vi "resolve VI reference.vi"(8 "error in":errorcluster, 10 "VI name":string, 11 "VI reference":refnum<vi>) -> (0 "error out":errorcluster, 3 "UI Ref":refnum<vi>)   [LabVIEW 2013, in "UI Reference runtime.lvclass"]
uses:
  UI Reference runtime.lvclass
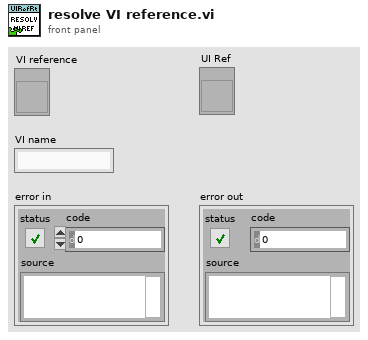
[diagram p1: front panel]
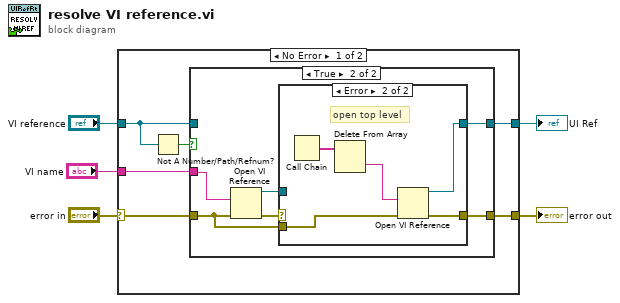
[diagram p0: block diagram]
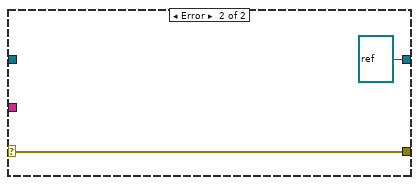
[diagram p4: hidden frame]
diagram:
  n1 = case shown="No Error" "error in" {
    selector: "error in" -> [w6 w28]
    tunnel: "VI reference" -> [w10 _]
    tunnel: [w9 refnum<vi> refnum ("VI reference")] -> w4
    tunnel: "VI name" -> [w8 _]
    tunnel: [w7 w28] -> w2
    frame No Error {
      n2 = Not A Number/Path/Refnum?(number/path/refnum=w10) -> (NaN/Path/Refnum?=w11:bool)
      n3 = case shown="True" w11 {
        tunnel: w10 -> [w13 _]
        tunnel: [w13 w17] -> w9
        tunnel: w6 -> [w12 w14]
        tunnel: w8 -> [_ w19]
        tunnel: [w12 w15] -> w7
        frame False {
        }
        frame True {
          n4 = Open VI Reference(vi path=w19, error in (no error)=w14) -> (vi reference=w16:refnum<vi>, error out=w18:errorcluster)  [unwired: 4 in]
          n5 = case shown="Error" w18 {
            selector: w18 -> [w20 _]
            tunnel: [w21 w24] -> w17
            tunnel: w16 -> [w21 _]
            tunnel: [w20 w25] -> w15
            tunnel: w14 -> [_ w26]
            frame No Error {
            }
            frame Error {
              # "open top level"
              n6 = Call Chain() -> (call chain=w23:string[])
              n7 = Delete From Array(array=w23) -> (deleted portion=w22:string)  [unwired: 2 in, 1 out]
              n8 = Open VI Reference(vi path=w22, error in (no error)=w26) -> (vi reference=w24:refnum<vi>, error out=w25:errorcluster)  [unwired: 4 in]
            }
          }
        }
      }
    }
    frame Error {
    }
  }
  "UI Ref" <- w4
  "error out" <- w2
